vi "Channel Names.vi"(8 "error in (no error)":errorcluster, 11 "Group in":refnum<class "Group.lvclass">) -> (0 "error out":errorcluster, 2 "Channel Names":string[](array[string]), 3 "Group out":refnum<class "Group.lvclass">)   [LabVIEW 2020, in "Vecto.lvlib" / "Group.lvclass"]
uses:
  Group.lvclass
  Group Config/Group Config.lvclass
  Channel Config/Channel Config.lvclass
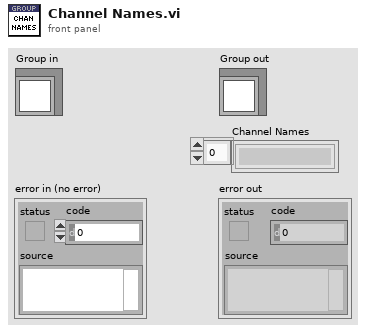
[diagram p1: front panel]
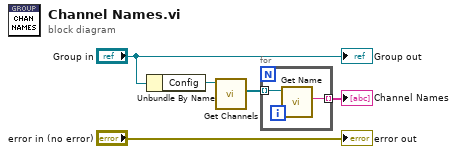
[diagram p0: block diagram]
diagram:
  n1 = Unbundle By Name("Group in") -> ("Config"=w3:refnum<class "Group Config.lvclass">)
  n2 = call "Get Channels.vi"("Group Config in"=w3) -> ("Channels"=w2:refnum<class "Channel Config.lvclass">[])  [unwired: 8 in, 2 out]
  n3 = for {
    tunnel: w2 -> [w7] mode=indexing
    tunnel: [w6] -> w1 mode=indexing
    n4 = call "Get Name.vi"("Channel Config in"=w7) -> ("Name"=w6:string)  [unwired: 8 in, 2 out]
  }
  "Channel Names" <- w1
  "error out" <- "error in (no error)"
  "Group out" <- "Group in"
